vi "writeToXML.vi"(8 "error in (no error)":errorcluster, 10 "classLabel":string, 11 "TargetConfiguration in":refnum<class "TargetConfiguration.lvclass">) -> (0 "error out":errorcluster, 2 "XML out":string, 3 "TargetConfiguration out":refnum<class "TargetConfiguration.lvclass">)   [LabVIEW 2022 SP3, in "TCSDataDefinitions.lvlib" / "TCSCommand.lvlib" / "TargetConfiguration.lvlib" / "TargetConfiguration.lvclass"]
uses:
  TargetConfiguration.lvclass
  <userlib>/Common/UnitsAndXML/FlattenItemWithUnitToXML/FlattenLengthToXML/LengthUnit.ctl
  TargetConfiguration.lvclass/TargetConfiguration.ctl
  TCSTcsCommand/TCSTcsCommand.lvclass
  Target/Target/Target.lvclass
  <userlib>/Common/UnitsAndXML/UnitsAndXML.lvlib
  <userlib>/Common/XML/XMLGenerator/XMLGenerator.lvclass
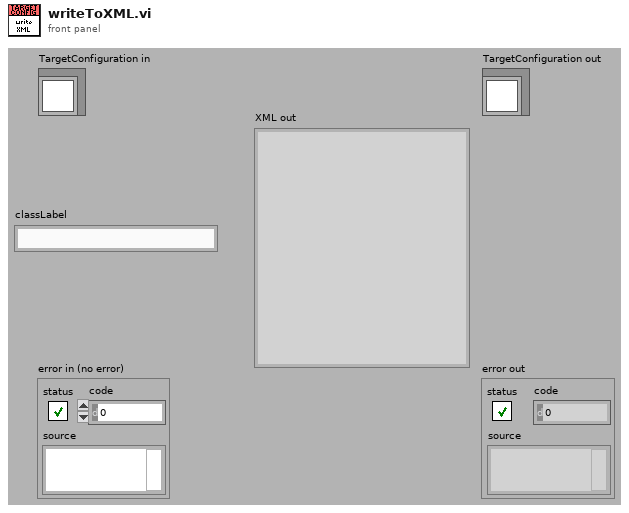
[diagram p1: front panel]
types:
  T1 = typedef "UnitsAndXML.lvlib/LengthUnit.ctl" = enum16{"m", "Angstrom", "AU", "chain", "cm", "cubit", "fathom", "fermi", "ft", "furlong", "hubble", "in", "ly", "mi", "mm", "rod", "um", "yd"}
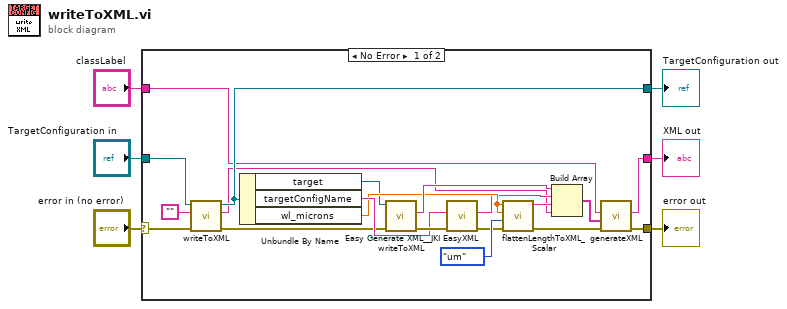
[diagram p0: block diagram]
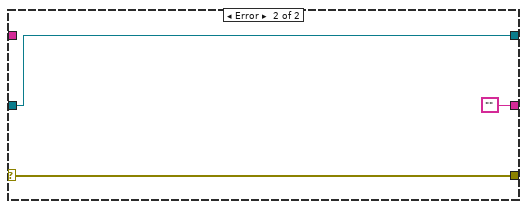
[diagram p2: hidden frame]
diagram:
  n1 = case shown="No Error" "error in (no error)" {
    selector: "error in (no error)" -> [w11 w29]
    tunnel: [w9 w29] -> w5
    tunnel: [w24 w28] -> w3
    tunnel: "TargetConfiguration in" -> [w26 w28]
    tunnel: [w12 ""] -> w2
    tunnel: "classLabel" -> [w10 _]
    frame No Error {
      n2 = call-parent "writeToXML.vi"("error in (no error)"=w11, "ClassLabel"="", "TCSTcsCommand in"=w26) -> ("error out"=w17:errorcluster, "XML out"=w8:string, "TCSTcsCommand out"=w24:refnum<class "TargetConfiguration.lvclass">)  [unwired: 6 in]
      n3 = Unbundle By Name(w24) -> ("target"=w7:refnum<class "Target.lvclass">, "targetConfigName"=w22:string, "wl_microns"=w20:dbl[unit])
      n4 = call-dynamic "writeToXML.vi"("error in (no error)"=w17, "Target in"=w7) -> ("error out"=w23:errorcluster, "XML out"=w21:string)  [unwired: 7 in, 1 out]
      n5 = call <vilib>:"Easy Generate XML__JKI EasyXML.vi"("error in (no error)"=w23, "LabVIEW Data"=w22) -> ("error out"=w18:errorcluster, "XML String"=w15:string)  [unwired: 8 in]
      n6 = call <userlib>:"flattenLengthToXML_Scalar.vi"("error in (no error)"=w18, "lengthUnitInXML"=LengthUnit."um", "lengthAgain"=w20, "length"=w20) -> ("error out"=w16:errorcluster, "xmlString"=w14:string)  [unwired: 6 in]
      n7 = Build Array(w21, w15, w14, w8) -> (w13:string[])
      n8 = call <userlib>:"generateXML.vi"("error in"=w16, "childrenXML"=w13, "elementName"=w10) -> ("error out"=w9:errorcluster, "XML out"=w12:string)  [unwired: 6 in, 1 out]
    }
    frame Error {
    }
  }
  "error out" <- w5
  "TargetConfiguration out" <- w3
  "XML out" <- w2
